vi "读信号循环发送参数文件.vi"(5 "error in (no error)":errorcluster caption="错误输入（无错误）") -> (14 "信号轮询发送设置Out":cluster{"XNET SignalFrameArry":T2[]}, 19 "error out":errorcluster caption="错误输出")   [LabVIEW 2020, in "ECU_Diagnose.lvlib" / "SignalSenderLoop.lvclass"]
uses:
  SignalSenderLoop.lvclass
  subvi/SignalFrameSet.ctl
  SignalReceiver/Typedefs/SignalArrySelecte.ctl
  <vilib>/Utility/config.llb/NI_LVConfig.lvlib
  SignalReceiver/SignalReceiver.lvclass
panel:
  in  "信号收发参数":T3={"信号接收参数"={"Port_No."="CAN1", "XNET Signal"=[]}, "信号轮询发送参数"={"XNET SignalFrameArry"=[{"Port_No."="CAN1", "计数Count"=TRUE, "校验CheckSum"=TRUE, "MessageFrame"="ESP_1\nLR110", "校验算法名称"="Anti_Add"}, {"Port_No."="CAN1", "计数Count"=FALSE, "校验CheckSum"=FALSE, "MessageFrame"="VTOG_1\nLR110", "校验算法名称"=""}]}}
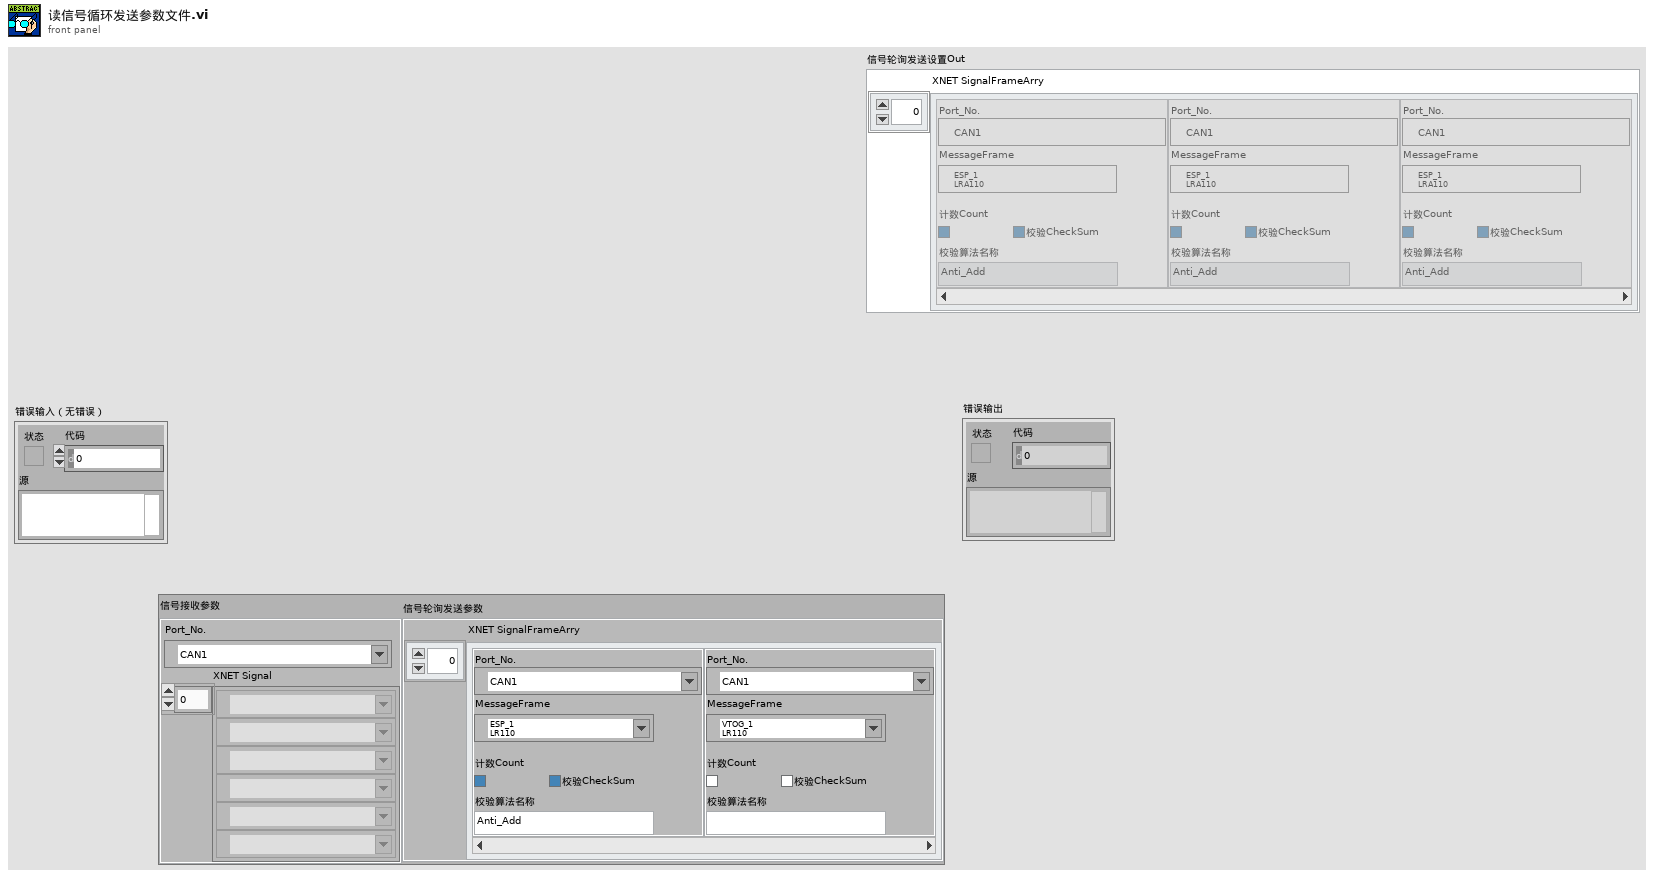
[diagram p1: front panel]
types:
  T1 = typedef "ECU_Diagnose.lvlib/SignalReceiver.lvclass/SignalArrySelecte.ctl" = cluster{"Port_No.":refnum<k21>, "XNET Signal":refnum<k21>[]}
  T2 = typedef "ECU_Diagnose.lvlib/SignalSenderLoop.lvclass/SignalFrameSet.ctl" = cluster{"Port_No.":refnum<k21>, "计数Count":bool, "校验CheckSum":bool, "MessageFrame":refnum<k21>, "校验算法名称":string}
  T3 = cluster{"信号接收参数":T1, "信号轮询发送参数":cluster{"XNET SignalFrameArry":T2[]}}
  T4 = typedef "NI_LVConfig.lvlib/Config Data RefNum.ctl" = refnum<k1>
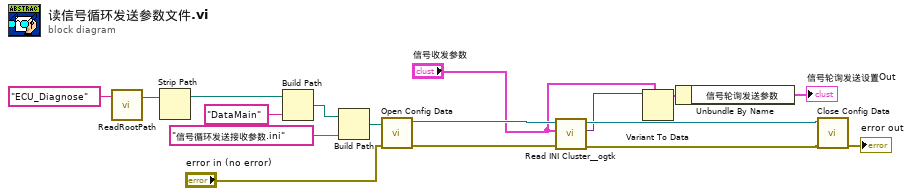
[diagram p0: block diagram]
diagram:
  n1 = call "ReadRootPath.vi"("BuildRootFolder"="ECU_Diagnose" ("ConfigFlieFolderName")) -> ("Root path"=w9:path)  [unwired: 18 in]
  n2 = Strip Path(path=w9) -> (stripped path=w8:path)  [unwired: 1 out]
  n3 = Build Path(base path=w8, name or relative path="DataMain" ("ConfigFlieFolderName")) -> (appended path=w14:path)
  n4 = Build Path(base path=w14, name or relative path="信号循环发送接收参数.ini" ("ConfigFlieFolderName")) -> (appended path=w13:path)
  n5 = call <vilib>:"Open Config Data.vi"("error in (no error)"="error in (no error)", "configuration file path"=w13) -> ("error out"=w6:errorcluster, "refnum"=w5:T4)  [unwired: 7 in, 1 out]
  n6 = call <userlib>:"Read INI Cluster__ogtk.vi"("error in (no error)"=w6, "INI Fomatted Cluster Type"="信号收发参数", "refnum"=w5) -> ("error out"=w16:errorcluster, "INI Fomatted Cluster"=w4:variant, "dup refnum"=w17:T4)  [unwired: 4 in, 2 out]
  n7 = Variant To Data(type="信号收发参数", Variant=w4) -> (data=w2:T3)  [unwired: 1 in, 1 out]
  n8 = Unbundle By Name(w2) -> ("信号轮询发送参数"=→"信号轮询发送设置Out":cluster{"XNET SignalFrameArry":T2[]})
  n9 = call <vilib>:"Close Config Data.vi"("error in (no error)"=w16, "refnum"=w17) -> ("error out"=→"error out":errorcluster)  [unwired: 8 in, 1 out]
